vi "MotorManager.vi"(3 "error in (no error)":errorcluster caption="错误输入（无错误）", 4 "Input":T2, 5 "ref_in":T1) -> (0 "error out":errorcluster caption="错误输出", 1 "Output":T2, 2 "ref_out":T1)   [LabVIEW 2012]
uses:
  D:/workspace/GitHub/LVsolis/AGUC2/AgilisCmdLib.dll
  AGUC2/AgilisCmdLib.dll
  D:/workspace/GitHub/LVsolis/lib/CmdLib.dll
  lib/CmdLib.dll
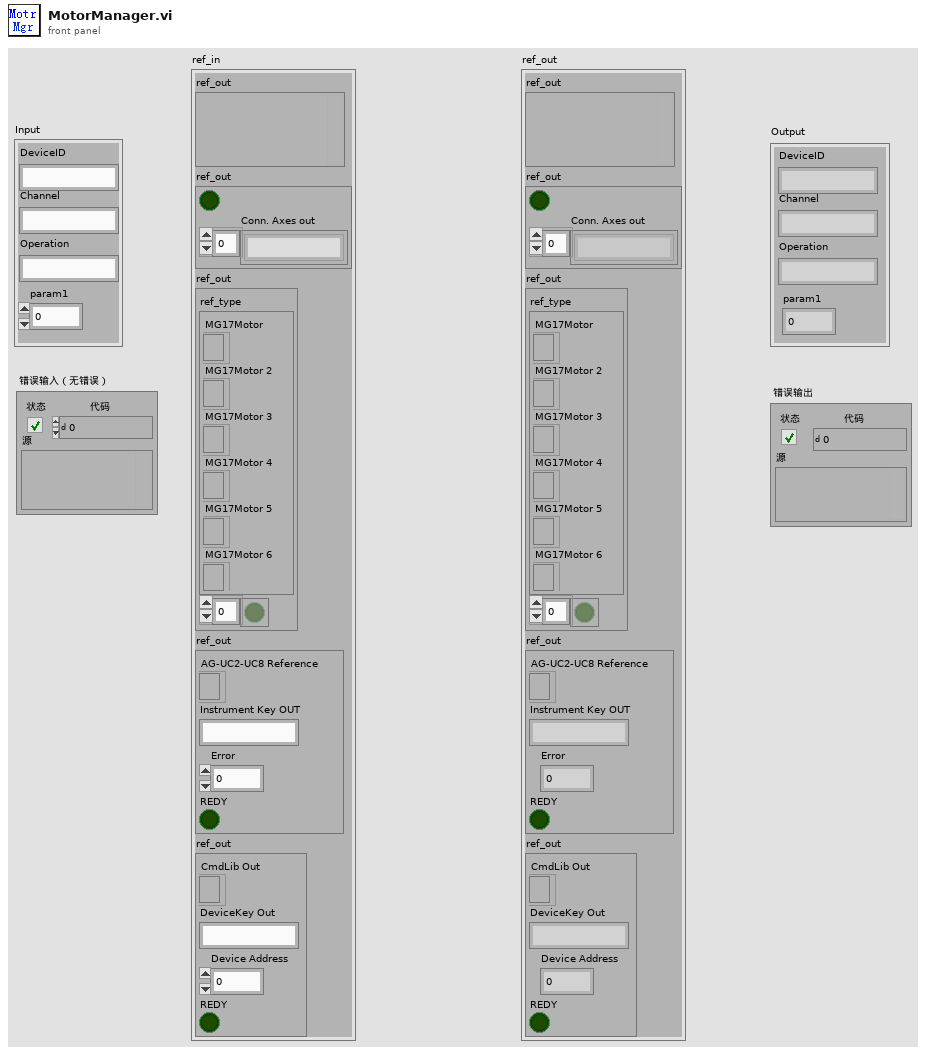
[diagram p1: front panel]
types:
  T1 = cluster{"ref_out":variant, "ref_out":cluster{bool, "Conn. Axes out":string[]}, "ref_out":cluster{"ref_type":cluster{"MG17Motor":refnum<k7>, "MG17Motor 2":refnum<k7>, "MG17Motor 3":refnum<k7>, "MG17Motor 4":refnum<k7>, "MG17Motor 5":refnum<k7>, "MG17Motor 6":refnum<k7>}, bool[]}, "ref_out":cluster{"AG-UC2-UC8 Reference":refnum<k24>, "Instrument Key OUT":string, "Error":i32, "REDY":bool}, "ref_out":cluster{"CmdLib Out":refnum<k24>, "DeviceKey Out":string, "Device Address":i32, "REDY":bool}}
  T2 = cluster{"DeviceID":string, "Channel":string, "param1":dbl, "Operation":string}
  T3 = cluster{"CmdLib Out":refnum<k24>, "DeviceKey Out":string, "Device Address":i32, "REDY":bool}
  T4 = cluster{"AG-UC2-UC8 Reference":refnum<k24>, "Instrument Key OUT":string, "Error":i32, "REDY":bool}
  T5 = cluster{"ref_type":cluster{"MG17Motor":refnum<k7>, "MG17Motor 2":refnum<k7>, "MG17Motor 3":refnum<k7>, "MG17Motor 4":refnum<k7>, "MG17Motor 5":refnum<k7>, "MG17Motor 6":refnum<k7>}, bool[]}
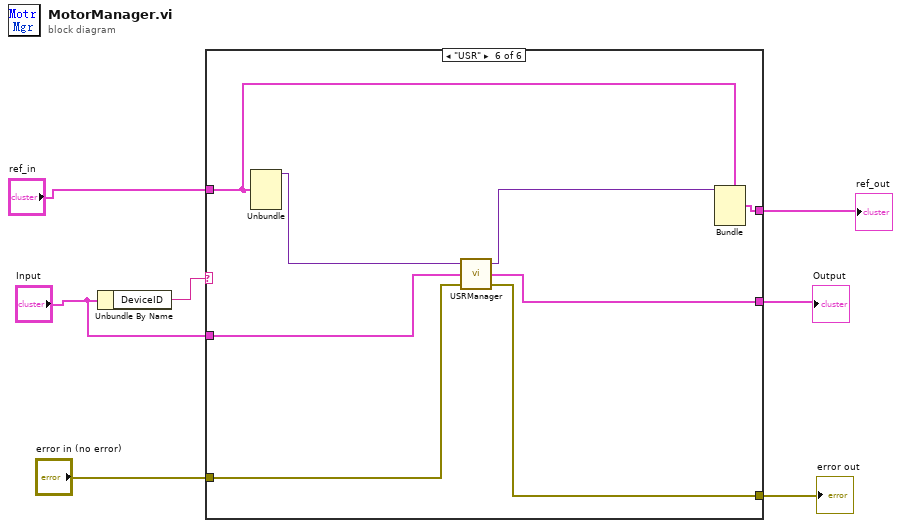
[diagram p0: block diagram]
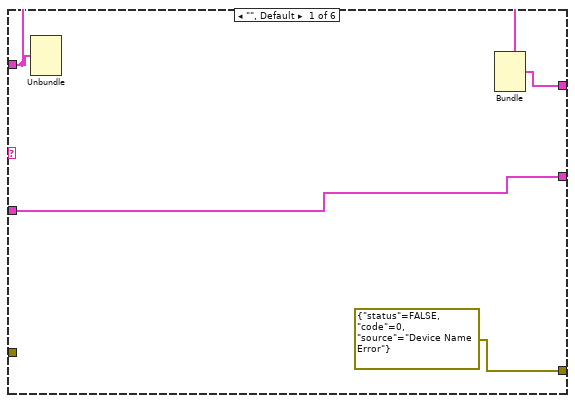
[diagram p2: hidden frame]
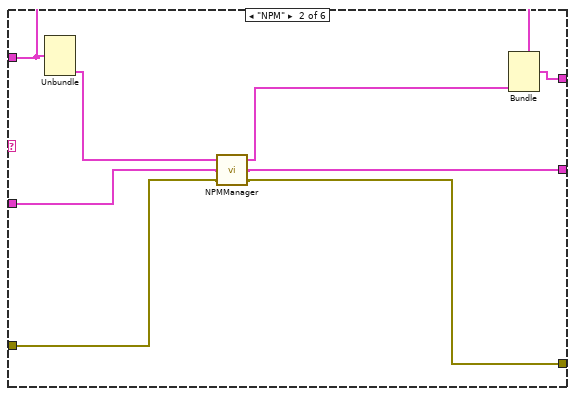
[diagram p3: hidden frame]
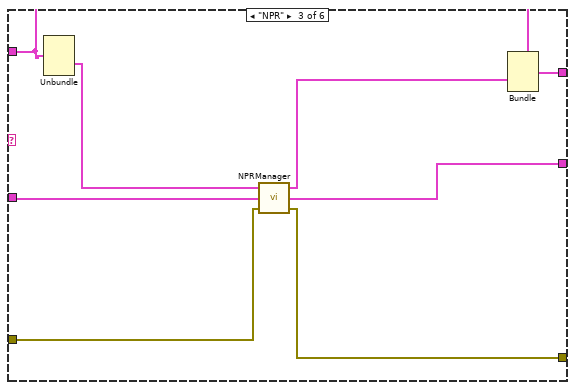
[diagram p4: hidden frame]
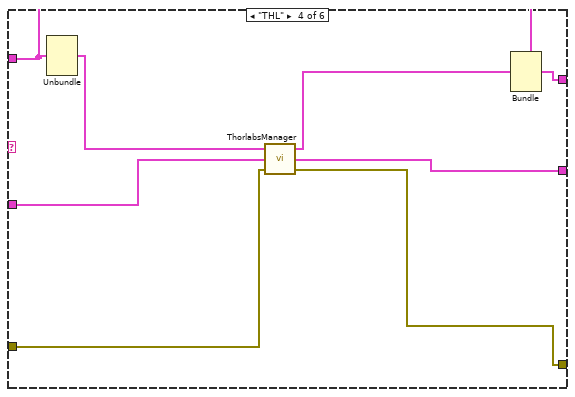
[diagram p5: hidden frame]
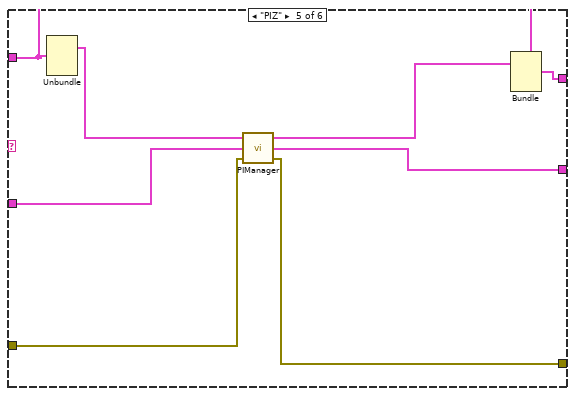
[diagram p6: hidden frame]
diagram:
  n1 = Unbundle By Name("Input") -> ("DeviceID"=w7:string)
  n2 = case shown="\"USR\"" w7 {
    tunnel: "Input" -> [w11 w16 w25 w33 w43 w49]
    tunnel: [w11 w17 w24 w32 w42 w48] -> w5
    tunnel: "error in (no error)" -> [_ w19 w27 w34 w41 w51]
    tunnel: [errorcluster {"status"=FALSE, "code"=0, "source"="Device Name Error"} ("error out") w18 w26 w35 w40 w50] -> w3
    tunnel: [w9 w14 w22 w30 w38 w46] -> w2
    tunnel: "ref_in" -> [w8 w15 w23 w31 w39 w47]
    frame "", Default {
      n3 = Unbundle(w8) -> ()  [unwired: 5 out]
      n4 = Bundle(cluster=w8) -> (w9:T1)  [unwired: 5 in]
    }
    frame "NPM" {
      n5 = Unbundle(w15) -> ("ref_out"=w13:T3)  [unwired: 4 out]
      n6 = call "NPMManager.vi"("error in (no error)"=w19, "Input"=w16, "ref_in"=w13) -> ("error out"=w18:errorcluster, "Output"=w17:T2, "ref_out"=w12:T3)
      n7 = Bundle(cluster=w15, "ref_out"=w12) -> (w14:T1)  [unwired: 4 in]
    }
    frame "NPR" {
      n8 = Unbundle(w23) -> ("ref_out"=w21:T4)  [unwired: 4 out]
      n9 = call "NPRManager.vi"("error in (no error)"=w27, "Input"=w25, "ref_in"=w21) -> ("error out"=w26:errorcluster, "Output"=w24:T2, "ref_out"=w20:T4)
      n10 = Bundle(cluster=w23, "ref_out"=w20) -> (w22:T1)  [unwired: 4 in]
    }
    frame "THL" {
      n11 = Unbundle(w31) -> ("ref_out"=w29:T5)  [unwired: 4 out]
      n12 = call "ThorlabsManager.vi"("error in (no error)"=w34, "Input"=w33, "ref_in"=w29) -> ("error out"=w35:errorcluster, "Output"=w32:T2, "ref_out"=w28:T5)
      n13 = Bundle(cluster=w31, "ref_out"=w28) -> (w30:T1)  [unwired: 4 in]
    }
    frame "PIZ" {
      n14 = Unbundle(w39) -> ("ref_out"=w37:cluster{bool, "Conn. Axes out":string[]})  [unwired: 4 out]
      n15 = call "PIManager.vi"("error in (no error)"=w41, "Input"=w43, "ref_in"=w37) -> ("error out"=w40:errorcluster, "Output"=w42:T2, "ref_out"=w36:cluster{bool, "Conn. Axes out":string[]})
      n16 = Bundle(cluster=w39, "ref_out"=w36) -> (w38:T1)  [unwired: 4 in]
    }
    frame "USR" {
      n17 = Unbundle(w47) -> ("ref_out"=w45:variant)  [unwired: 4 out]
      n18 = call "USRManager.vi"("error in (no error)"=w51, "Input"=w49, "ref_in"=w45) -> ("error out"=w50:errorcluster, "Output"=w48:T2, "ref_out"=w44:variant)
      n19 = Bundle(cluster=w47, "ref_out"=w44) -> (w46:T1)  [unwired: 4 in]
    }
  }
  "error out" <- w3
  "Output" <- w5
  "ref_out" <- w2
